vi "initCSMs.vi"(7 "Enable building lvlibp?":bool, 8 "error in (no error)":errorcluster, 11 "TestCase in":refnum<class "testcase-CSMGlobalLog.lvclass">) -> (0 "error out":errorcluster, 3 "TestCase out":refnum<class "testcase-CSMGlobalLog.lvclass">)   [LabVIEW 2017, in "testcase-CSMGlobalLog.lvclass"]
uses:
  testcase-CSMGlobalLog.lvclass
  CSM/Chain1.vi
  CSM/Chain2.vi
  CSM/Chain3.vi
  CSM/Normal-CSM.vi
  <vilib>/AppBuilder/AB_API_Simple/Build (path).vi
  CSM/CSM-Testcase.lvlib
  src/user.lib/_NEVSTOP/Communicable State Machine(CSM)/Communicable State Machine.lvlib
  <vilib>/AppBuilder/AB_API_Simple/NI_App_Builder_API.lvlib
panel:
  out "Waited (ms)":u32
  out "CSMs Left":string[](array[string])
  out "CSMs":string[](array[string])
  out "Generated files":path[](array[path])
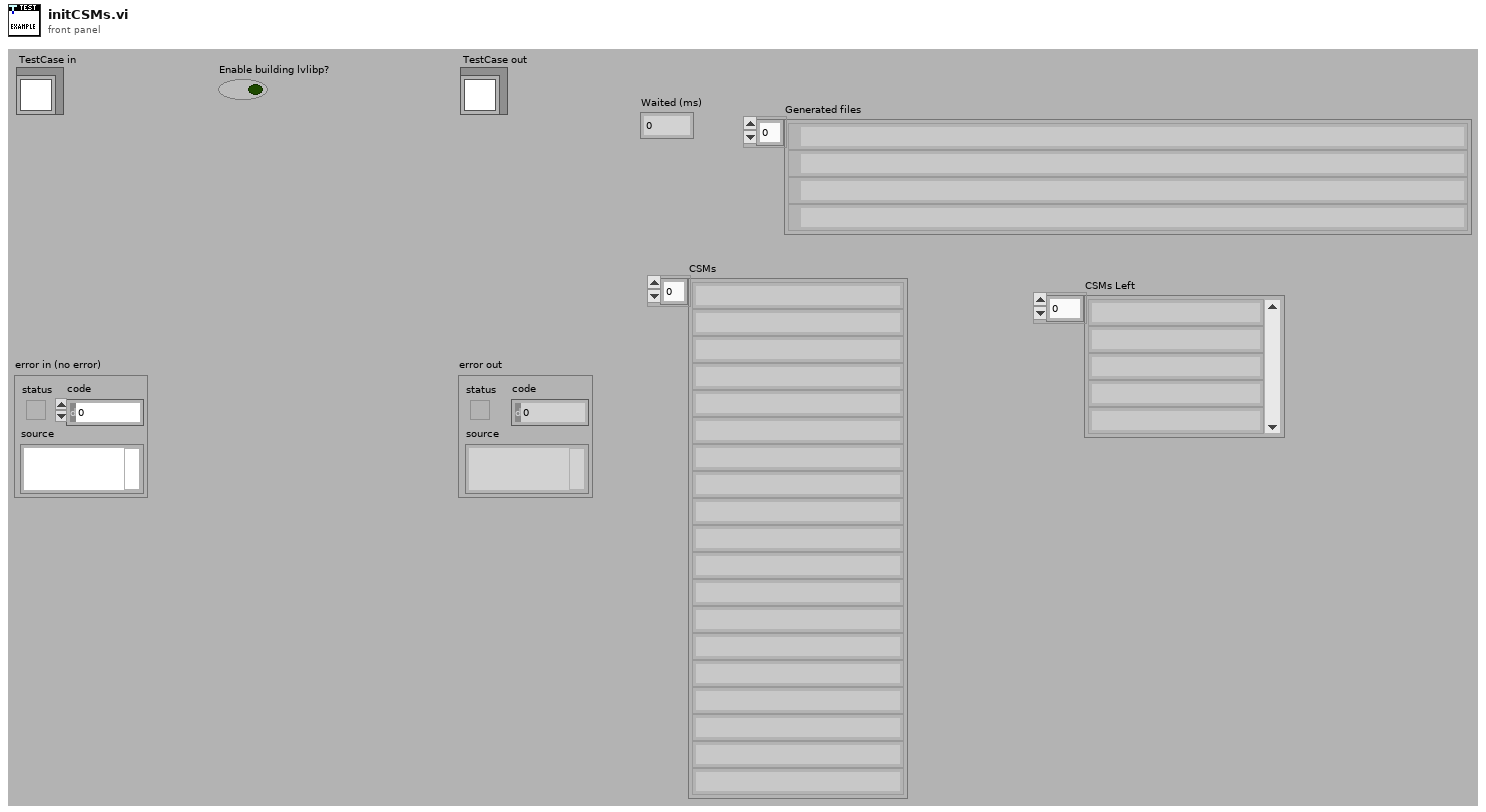
[diagram p1: front panel]
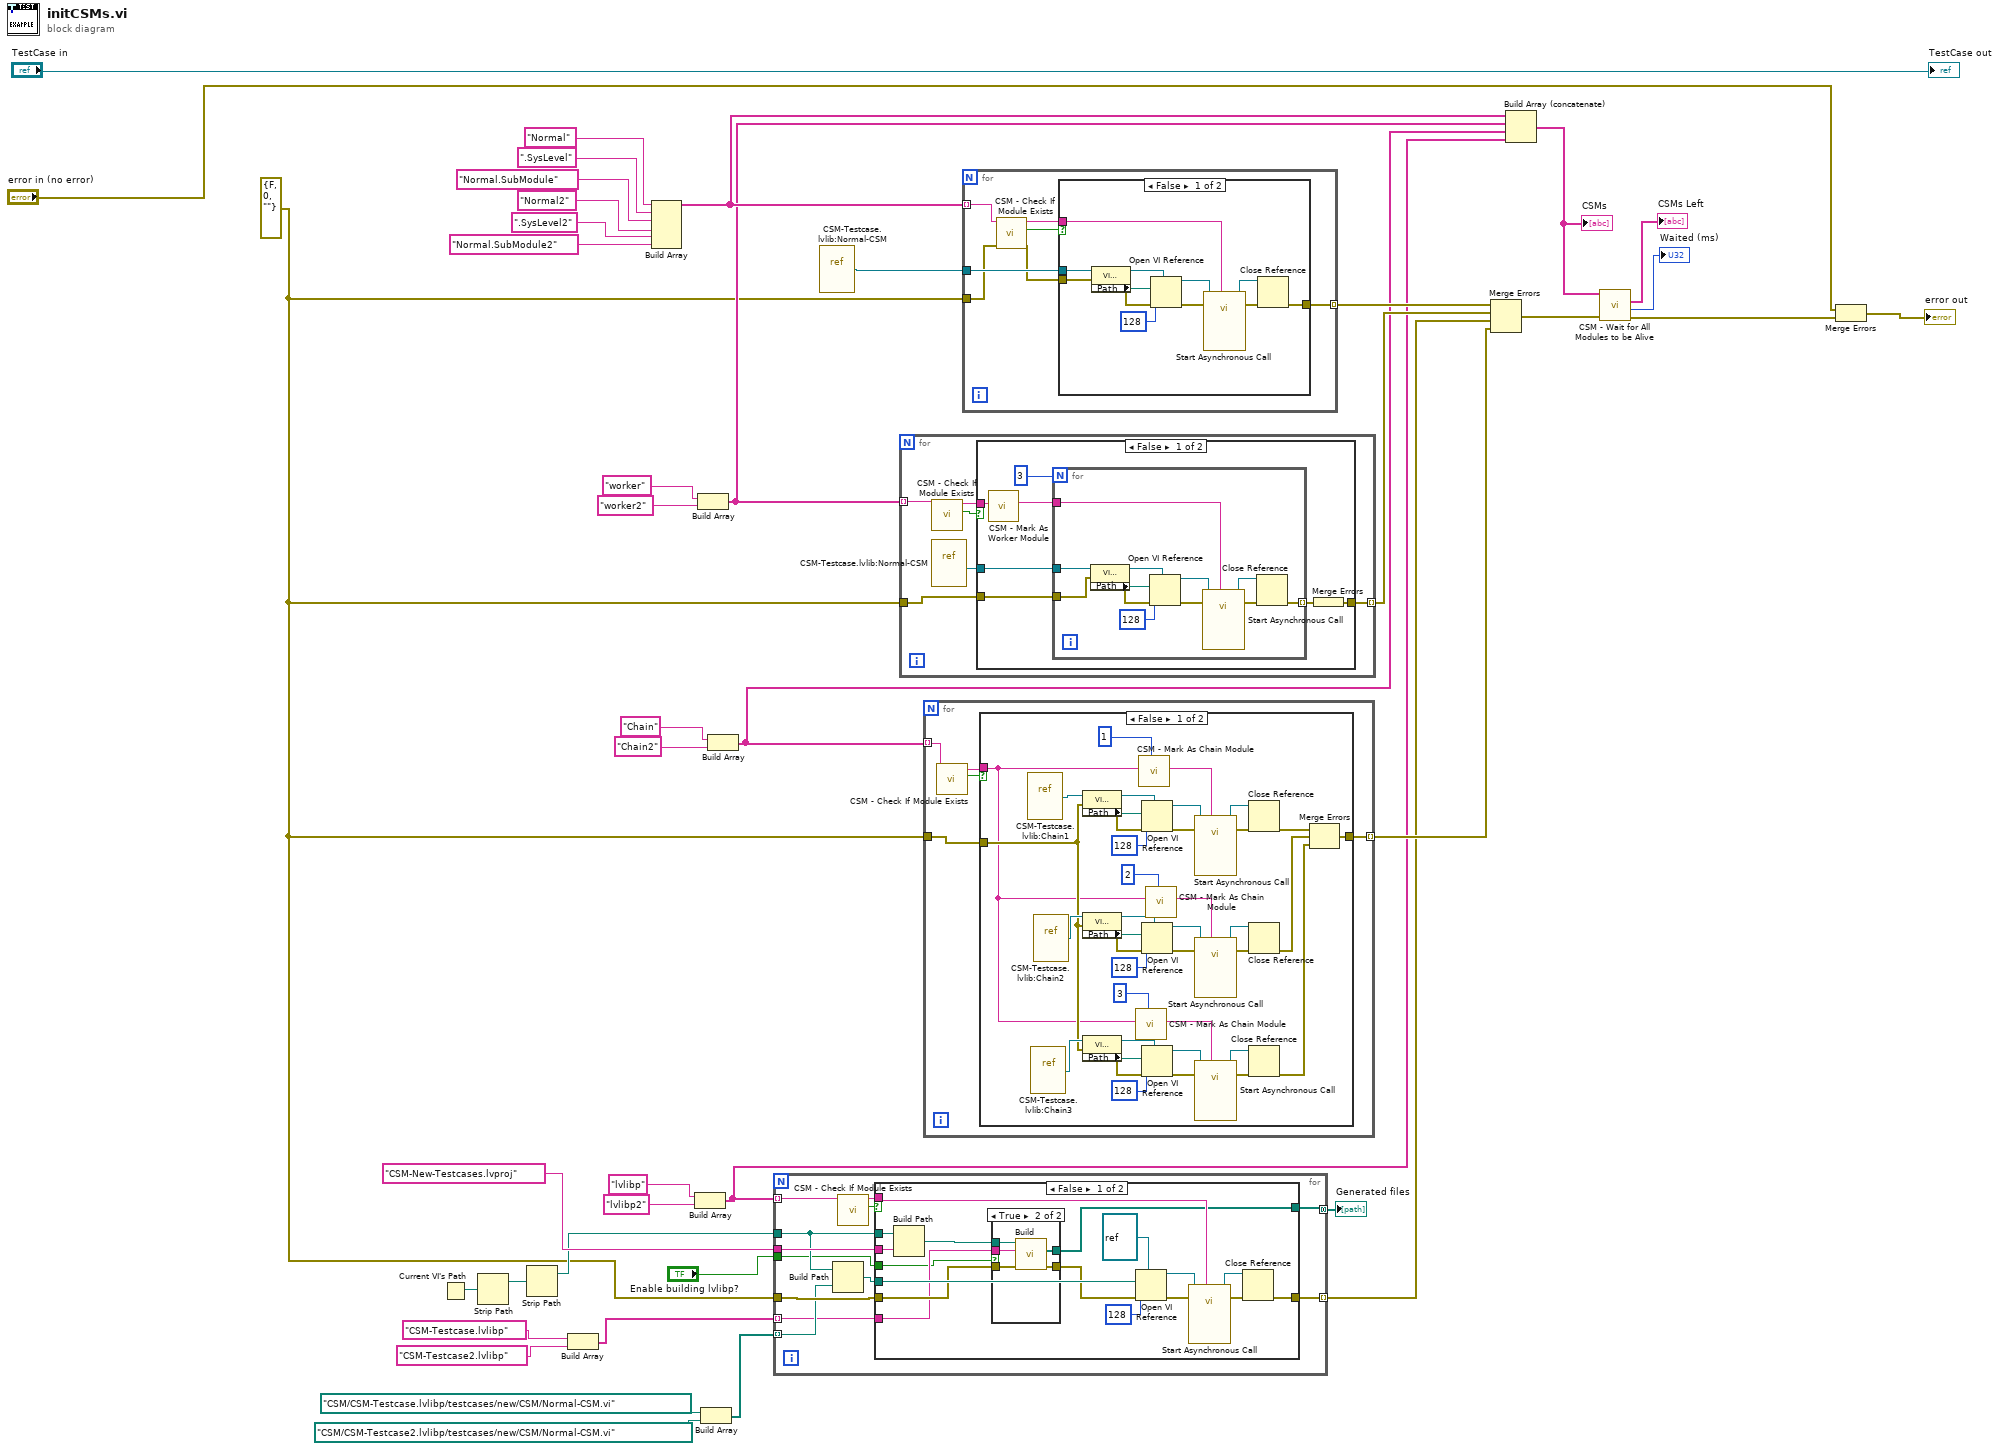
[diagram p0: block diagram]
diagram:
  w3 = errorcluster {"status"=FALSE, "code"=0, "source"=""} ("error in (no error)")
  n1 = Current VI's Path() -> (path=w38:path)
  n2 = Strip Path(path=w38) -> (stripped path=w39:path)  [unwired: 1 out]
  n3 = Strip Path(path=w39) -> (stripped path=w40:path)  [unwired: 1 out]
  n4 = Build Array("CSM-Testcase.lvlibp" ("Name of build specification (if empty: build all)"), "CSM-Testcase2.lvlibp" ("Name of build specification (if empty: build all)")) -> (w12:string[])
  n5 = Build Array("Normal" ("Name (\"\" to Use UUID)"), ".SysLevel" ("Name (\"\" to Use UUID)"), "Normal.SubModule" ("Name (\"\" to Use UUID)"), "Normal2" ("Name (\"\" to Use UUID)"), ".SysLevel2" ("Name (\"\" to Use UUID)"), "Normal.SubModule2" ("Name (\"\" to Use UUID)")) -> (w34:string[])
  n6 = Build Array("lvlibp" ("Name (\"\" to Use UUID)"), "lvlibp2" ("Name (\"\" to Use UUID)")) -> (w18:string[])
  n7 = Build Array("worker" ("Name (\"\" to Use UUID)"), "worker2" ("Name (\"\" to Use UUID)")) -> (w24:string[])
  n8 = Build Array(path "CSM/CSM-Testcase.lvlibp/testcases/new/CSM/Normal-CSM.vi" ("vi path"), path "CSM/CSM-Testcase2.lvlibp/testcases/new/CSM/Normal-CSM.vi" ("vi path")) -> (w15:path[])
  n9 = Build Array("Chain" ("Name (\"\" to Use UUID)"), "Chain2" ("Name (\"\" to Use UUID)")) -> (w21:string[])
  n10 = for {
    tunnel: "CSM-New-Testcases.lvproj" ("name or relative path") -> [w52]
    tunnel: w40 -> [w47]
    tunnel: w18 -> [w49] mode=indexing
    tunnel: w15 -> [w48] mode=indexing
    tunnel: w12 -> [w45] mode=indexing
    tunnel: [w44] -> w11 mode=concatenating
    tunnel: "Enable building lvlibp?" -> [w43]
    tunnel: w3 -> [w53]
    tunnel: [w51] -> w37 mode=indexing
    n11 = Build Path(base path=w47, name or relative path=w48) -> (appended path=w46:path)
    n12 = call "CSM - Check If Module Exists.vi"("CSM Name"=w49) -> ("Exist?"=w54:bool, "CSM Name (Dup)"=w50:string)  [unwired: 8 in, 1 out]
    n13 = case shown="False" w54 {
      tunnel: [w71 w78] -> w51
      tunnel: w46 -> [w64 _]
      tunnel: w47 -> [w63 _]
      tunnel: w52 -> [w61 _]
      tunnel: w50 -> [w60 _]
      tunnel: w53 -> [w59 w78]
      tunnel: w45 -> [w57 _]
      tunnel: [w56 _] -> w44
      tunnel: w43 -> [w55 _]
      frame False {
        n14 = Build Path(base path=w63, name or relative path=w61) -> (appended path=w62:path)
        n15 = case shown="True" w55 {
          tunnel: w62 -> [_ w77]
          tunnel: w59 -> [w72 w76]
          tunnel: [w72 w75] -> w58
          tunnel: w57 -> [_ w74]
          tunnel: [_ w73] -> w56
          frame False {
          }
          frame True {
            n16 = call-poly <vilib>:"Build.vi"("error in (no error)"=w76, "Name of build specification (if empty: build all)"=w74, "Path to project"=w77) -> ("error out"=w75:errorcluster, "Generated files"=w73:path[])  [unwired: 7 in]
          }
        }
        n17 = Open VI Reference(type specifier VI Refnum (for type only)=refnum<vi> refnum ("reference out"), vi path=w64, options=128, error in (no error)=w58) -> (vi reference=w67:refnum<vi>, error out=w69:errorcluster)  [unwired: 2 in]
        n18 = call-by-ref "Start Asynchronous Call"(reference=w67, error in=w69, "Name (\"\" to Use UUID)"=w60) -> (reference out=w66:refnum<vi>, error out=w68:errorcluster)  [unwired: 11 in]
        n19 = Close Reference(reference=w66, error in (no error)=w68) -> (error out=w71:errorcluster)
      }
      frame True {
      }
    }
  }
  "Generated files" <- w11
  n20 = vi-ref "CSM-Testcase.lvlib:Normal-CSM.vi"() -> (w30:refnum<vi>)
  n21 = for {
    tunnel: w24 -> [w79] mode=indexing
    tunnel: w3 -> [w84]
    tunnel: [w81] -> w36 mode=indexing
    n22 = call "CSM - Check If Module Exists.vi"("CSM Name"=w79) -> ("Exist?"=w83:bool, "CSM Name (Dup)"=w82:string)  [unwired: 8 in, 1 out]
    n23 = vi-ref "CSM-Testcase.lvlib:Normal-CSM.vi"() -> (w80:refnum<vi>)
    n24 = case shown="False" w83 {
      tunnel: w80 -> [w91 _]
      tunnel: [w85 w104] -> w81
      tunnel: w84 -> [w87 w104]
      tunnel: w82 -> [w86 _]
      frame False {
        n25 = call "CSM - Mark As Worker Module.vi"("CSM Name"=w86) -> ("CSM Name (Marked As Worker)"=w88:string)  [unwired: 9 in]
        n26 = for {
          N: 3 -> [_]
          tunnel: w91 -> [w95]
          tunnel: w88 -> [w94]
          tunnel: [w93] -> w89 mode=indexing
          tunnel: w87 -> [w92]
          n27 = property class="VI (strict)"(reference=w95, error in=w92) -> (reference out=w101:refnum<vi>, error out=w99:errorcluster, "Path"=w98:path)
          n28 = Open VI Reference(type specifier VI Refnum (for type only)=w101, vi path=w98, options=128, error in (no error)=w99) -> (vi reference=w97:refnum<vi>, error out=w102:errorcluster)  [unwired: 2 in]
          n29 = call-by-ref "Start Asynchronous Call"(reference=w97, error in=w102, "Name (\"\" to Use UUID)"=w94) -> (reference out=w96:refnum<vi>, error out=w100:errorcluster)  [unwired: 11 in]
          n30 = Close Reference(reference=w96, error in (no error)=w100) -> (error out=w93:errorcluster)
        }
        n31 = Merge Errors(w89) -> (w85:errorcluster)
      }
      frame True {
      }
    }
  }
  n32 = for {
    tunnel: w21 -> [w105] mode=indexing
    tunnel: w3 -> [w109]
    tunnel: [w107] -> w42 mode=indexing
    n33 = call "CSM - Check If Module Exists.vi"("CSM Name"=w105) -> ("Exist?"=w108:bool, "CSM Name (Dup)"=w106:string)  [unwired: 8 in, 1 out]
    n34 = case shown="False" w108 {
      tunnel: [w112 w149] -> w107
      tunnel: w109 -> [w111 w149]
      tunnel: w106 -> [w110 _]
      frame False {
        n35 = vi-ref "CSM-Testcase.lvlib:Chain1.vi"() -> (w148:refnum<vi>)
        n36 = vi-ref "CSM-Testcase.lvlib:Chain3.vi"() -> (w130:refnum<vi>)
        n37 = vi-ref "CSM-Testcase.lvlib:Chain2.vi"() -> (w131:refnum<vi>)
        n38 = property class="VI (strict)"(reference=w148, error in=w111) -> (reference out=w145:refnum<vi>, error out=w143:errorcluster, "Path"=w142:path)
        n39 = property class="VI (strict)"(reference=w131, error in=w111) -> (reference out=w134:refnum<vi>, error out=w136:errorcluster, "Path"=w137:path)
        n40 = property class="VI (strict)"(reference=w130, error in=w111) -> (reference out=w127:refnum<vi>, error out=w125:errorcluster, "Path"=w124:path)
        n41 = call "CSM - Mark As Chain Module.vi"("Order"=3, "CSM Name"=w110) -> ("CSM Name (Marked As Chain)"=w118:string)  [unwired: 8 in]
        n42 = call "CSM - Mark As Chain Module.vi"("Order"=1, "CSM Name"=w110) -> ("CSM Name (Marked As Chain)"=w116:string)  [unwired: 8 in]
        n43 = Open VI Reference(type specifier VI Refnum (for type only)=w145, vi path=w142, options=128, error in (no error)=w143) -> (vi reference=w141:refnum<vi>, error out=w146:errorcluster)  [unwired: 2 in]
        n44 = Open VI Reference(type specifier VI Refnum (for type only)=w134, vi path=w137, options=128, error in (no error)=w136) -> (vi reference=w138:refnum<vi>, error out=w133:errorcluster)  [unwired: 2 in]
        n45 = Open VI Reference(type specifier VI Refnum (for type only)=w127, vi path=w124, options=128, error in (no error)=w125) -> (vi reference=w123:refnum<vi>, error out=w128:errorcluster)  [unwired: 2 in]
        n46 = call "CSM - Mark As Chain Module.vi"("Order"=2, "CSM Name"=w110) -> ("CSM Name (Marked As Chain)"=w117:string)  [unwired: 8 in]
        n47 = call-by-ref "Start Asynchronous Call"(reference=w141, error in=w146, "Name (\"\" to Use UUID)"=w116) -> (reference out=w140:refnum<vi>, error out=w144:errorcluster)  [unwired: 11 in]
        n48 = call-by-ref "Start Asynchronous Call"(reference=w138, error in=w133, "Name (\"\" to Use UUID)"=w117) -> (reference out=w139:refnum<vi>, error out=w135:errorcluster)  [unwired: 11 in]
        n49 = call-by-ref "Start Asynchronous Call"(reference=w123, error in=w128, "Name (\"\" to Use UUID)"=w118) -> (reference out=w122:refnum<vi>, error out=w126:errorcluster)  [unwired: 11 in]
        n50 = Close Reference(reference=w140, error in (no error)=w144) -> (error out=w121:errorcluster)
        n51 = Close Reference(reference=w139, error in (no error)=w135) -> (error out=w120:errorcluster)
        n52 = Close Reference(reference=w122, error in (no error)=w126) -> (error out=w119:errorcluster)
        n53 = Merge Errors(w121, w120, w119) -> (w112:errorcluster)
      }
      frame True {
      }
    }
  }
  n54 = for {
    tunnel: w30 -> [w156]
    tunnel: w34 -> [w152] mode=indexing
    tunnel: [w155] -> w35 mode=indexing
    tunnel: w3 -> [w154]
    n55 = call "CSM - Check If Module Exists.vi"("Error In"=w154, "CSM Name"=w152) -> ("error out"=w153:errorcluster, "Exist?"=w150:bool, "CSM Name (Dup)"=w151:string)  [unwired: 7 in]
    n56 = case shown="False" w150 {
      tunnel: w156 -> [w160 _]
      tunnel: [w159 w169] -> w155
      tunnel: w153 -> [w158 w169]
      tunnel: w151 -> [w157 _]
      frame False {
        n57 = property class="VI (strict)"(reference=w160, error in=w158) -> (reference out=w166:refnum<vi>, error out=w164:errorcluster, "Path"=w163:path)
        n58 = Open VI Reference(type specifier VI Refnum (for type only)=w166, vi path=w163, options=128, error in (no error)=w164) -> (vi reference=w162:refnum<vi>, error out=w167:errorcluster)  [unwired: 2 in]
        n59 = call-by-ref "Start Asynchronous Call"(reference=w162, error in=w167, "Name (\"\" to Use UUID)"=w157) -> (reference out=w161:refnum<vi>, error out=w165:errorcluster)  [unwired: 11 in]
        n60 = Close Reference(reference=w161, error in (no error)=w165) -> (error out=w159:errorcluster)
      }
      frame True {
      }
    }
  }
  n61 = Merge Errors(w35, w36, w37, w42) -> (w10:errorcluster)
  n62 = Build Array (concatenate)(w34, w24, w21, w18) -> (w9:string[])
  "CSMs" <- w9
  n63 = call "CSM - Wait for All Modules to be Alive.vi"("Error In"=w10, "CSM Names"=w9) -> ("error out"=w5:errorcluster, "Waited (ms)"=→"Waited (ms)":u32, "CSMs Left"=→"CSMs Left":string[])  [unwired: 7 in]
  n64 = Merge Errors("error in (no error)", w5) -> (→"error out":errorcluster)
  "TestCase out" <- "TestCase in"
